vi "Joud_signal_generation.vi"() -> ()   [LabVIEW 2020]
uses:
  <vilib>/Utility/file.llb/Read Delimited Spreadsheet (DBL).vi
panel:
  in  "Scale":dbl
  out "first row":dbl[](array[numeric])
  out "Input":waveform(dbl)(graph)
  in  "file to run":path=path "C:/Users/Puja/Desktop/Labview(PC)/Input_Signal/Sine_wave_data_without_time/data1_w1_NT_1per.txt"
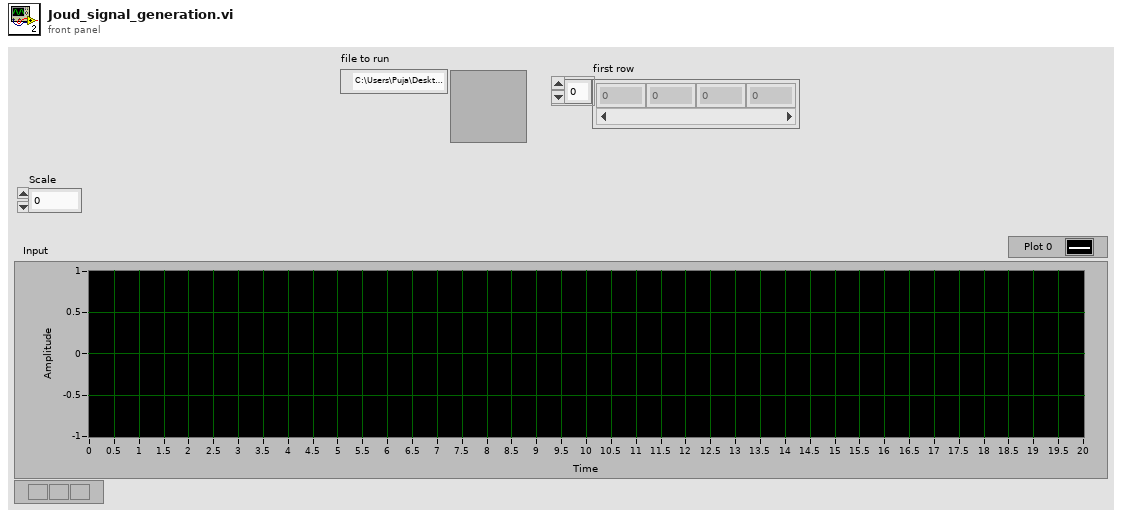
[diagram p1: front panel]
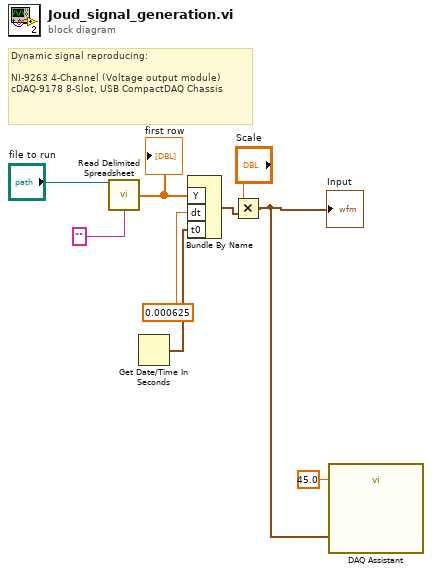
[diagram p0: block diagram]
diagram:
  # "Dynamic signal reproducing:\n\nNI-9263 4-Channel (Voltage output module)\ncDAQ-9178 8-Slot, USB CompactDAQ Chassis"
  n1 = call-poly <vilib>:"Read Delimited Spreadsheet.vi"("file path (dialog if empty)"="file to run", "delimiter (\\t)"="") -> ("first row"=w8:dbl[])  [unwired: 8 in, 5 out]
  "first row" <- w8
  n2 = Get Date/Time In Seconds() -> (seconds since 1Jan1904=w6:timestamp)
  n3 = Bundle By Name("Y"=w8, "dt"=0.000625, "t0"=w6) -> (w4:waveform(dbl))  [unwired: 1 in]
  n4 = Multiply(x="Scale", y=w4) -> (x*y=w2:waveform(dbl))
  "Input" <- w2
  n5 = call "DAQ Assistant"("data"=w2, "timeout (s)"=45.0) -> ()  [unwired: 16 in, 2 out]
